vi "Mutex Timed Lock (absolute seconds).vi"(8 "error in (no error)":errorcluster, 10 "absolute timeout (seconds)":dbl, 11 "Mutex in":T1) -> (0 "error out":errorcluster, 2 "timed out?":bool, 3 "Mutex out":T1)   [LabVIEW 2013, in "POSIX Threads.lvlib" / "Mutex.lvclass"]
doc: "Calls pthread_mutex_timedlock() on the pthread mutex object encapsulated by Mutex.\n\nThis VI attempts to lock the provided mutex in a specified timeout period. To provide a valid absolute timeout, query the Realtime clock for the current time and offset the time by the desired timeout duration.\n\nRefer to online POSIX documentation for more information."
uses:
  Mutex.lvclass
  Controls/reference.ctl
  POSIX Thread Object/POSIX Thread Object.lvclass/POSIX Thread Object.ctl
  POSIX Thread Object/Private VIs/libpthread path.vi
  <vilib>/NI/NI Linux RT Utilities/VIs/Public/Convert Types/convert timespec 64 to timespec 32.vi
  POSIX Thread Object/Private VIs/get pthread error.vi
  POSIX Thread Object/POSIX Thread Object.lvclass
  <vilib>/NI/NI Linux RT Utilities/Linux RT Utilities.lvlib
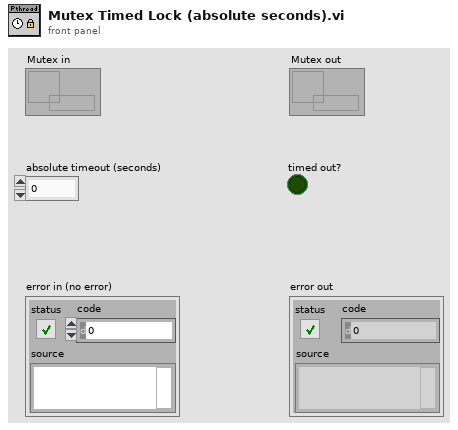
[diagram p1: front panel]
types:
  T1 = typedef "POSIX Threads.lvlib/Mutex.lvclass/reference.ctl" = refnum<data-value>
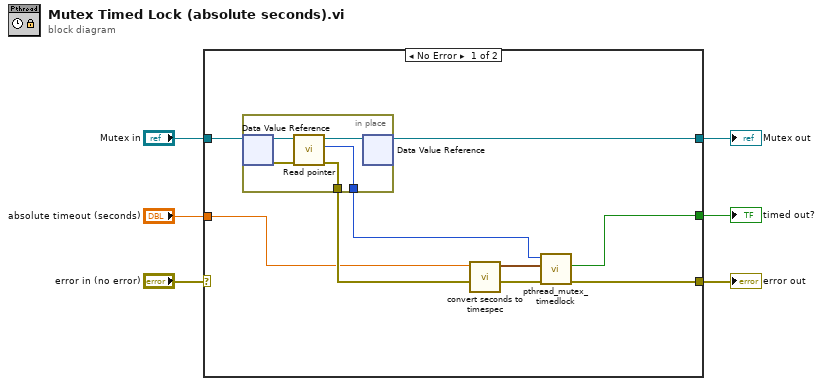
[diagram p0: block diagram]
diagram:
  n1 = case shown="No Error" "error in (no error)" {
    selector: "error in (no error)" -> [_ w21]
    tunnel: [w14 w21] -> w5
    tunnel: "Mutex in" -> [w11 w20]
    tunnel: [w10 w20] -> w3
    tunnel: "absolute timeout (seconds)" -> [w7 _]
    tunnel: [w13 _] -> w1
    frame No Error {
      n2 = in-place {
        in-place-border: [w16] -> w8
        in-place-border: [w15] -> w9
        n3 = in-place-dvr #1(w11) -> (w19:refnum<class "Mutex.lvclass">, w17:errorcluster)
        n4 = call "Read pointer.vi"("error in (no error)"=w17, "POSIX Thread Object in"=w19) -> ("error out"=w16:errorcluster, "pointer"=w15:u64, "POSIX Thread Object out"=w18:refnum<class "Mutex.lvclass">)  [unwired: 7 in]
        n5 = in-place-dvr #1(w18) -> (w10:T1)  [unwired: 1 out]
      }
      n6 = call <vilib>:"convert seconds to timespec.vi"("seconds"=w7) -> ("timespec"=w12:cluster{"sec":u64, "nsec":u64})  [unwired: 10 in]
      n7 = call "pthread_mutex_timedlock.vi"("error in (no error)"=w8, "absolute time"=w12, "mutex ptr in"=w9) -> ("error out"=w14:errorcluster, "timed out?"=w13:bool)  [unwired: 6 in, 1 out]
    }
    frame Error {
    }
  }
  "Mutex out" <- w3
  "error out" <- w5
  "timed out?" <- w1
